vi "Simulated VeriStand Engine.Interface.Get Control Pointers.vi"(8 "error in (no error)":errorcluster, 11 "Simulated VeriStand Engine Interface in":refnum<class "Simulated VeriStand Engine.Interface.lvclass">) -> (0 "error out":errorcluster, 2 "Control Pointers":T1, 3 "Simulated VeriStand Engine Interface out":refnum<class "Simulated VeriStand Engine.Interface.lvclass">)   [LabVIEW 2016, in "Simulated VeriStand Engine.Interface.lvclass"]
uses:
  Simulated VeriStand Engine.Interface.lvclass
  Typedefs/Simulated VeriStand Engine.Interface.Pointers.Control.ctl
  Source/Submodules/Memory/Source/Classes/Internal/Memory.Pointer.Internal.lvclass
  Simulated VeriStand Engine.Interface.lvclass/Simulated VeriStand Engine.Interface.ctl
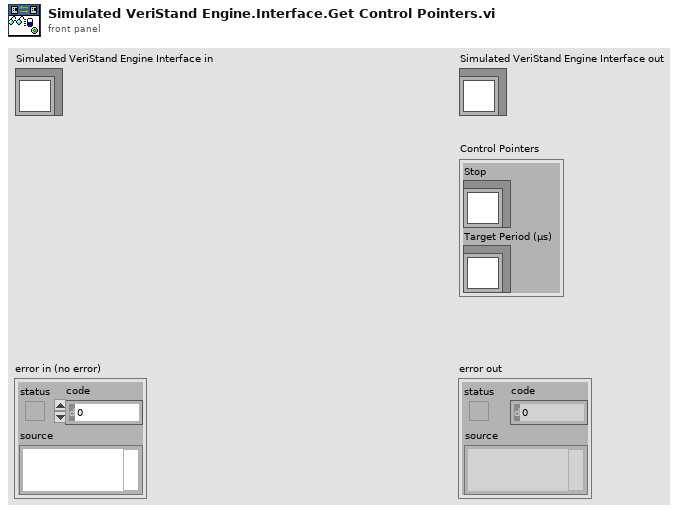
[diagram p1: front panel]
types:
  T1 = typedef "Simulated VeriStand Engine.Interface.lvclass/Simulated VeriStand Engine.Interface.Pointers.Control.ctl" = cluster{"Stop":refnum<class "Memory.Pointer.Internal.lvclass">, "Target Period (µs)":refnum<class "Memory.Pointer.Internal.lvclass">}
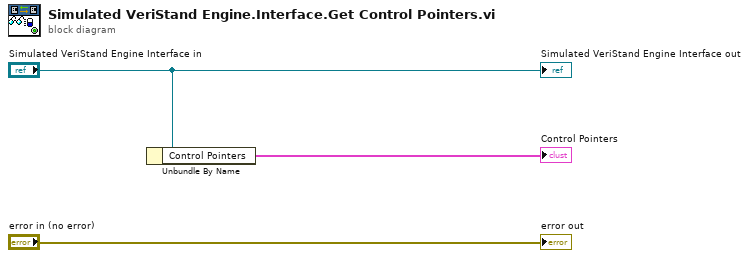
[diagram p0: block diagram]
diagram:
  n1 = Unbundle By Name("Simulated VeriStand Engine Interface in") -> ("Control Pointers"=→"Control Pointers":T1)
  "error out" <- "error in (no error)"
  "Simulated VeriStand Engine Interface out" <- "Simulated VeriStand Engine Interface in"
